vi "Receive Messages.vi"(6 "Wait Time":i32=-1, 8 "error in (no error)":errorcluster, 9 "Visibility Timeout":i32, 10 "Max Number of Messages":i32=1, 11 "SQS in":refnum<class "Queue.lvclass">) -> (0 "error out":errorcluster, 2 "Messages":T1[](array[typedef]), 3 "SQS out":refnum<class "Queue.lvclass">)   [LabVIEW 2015, in "NI_AWS_SQS.lvlib" / "Queue.lvclass"]
doc: "Retrieves one or more messages (up to 10), from the specified queue. Using the Wait Time parameter enables long-poll support. For more information, see Amazon SQS Long Polling in the Amazon SQS Developer Guide.\n\nShort poll is the default behavior where a weighted random set of machines is sampled on a ReceiveMessage call. Thus, only the messages on the sampled machines are returned. If the number of messages in the queue is small (fewer than 1,000), you most likely get fewer messages than you requested per ReceiveMessage call. If the number of messages in the queue is extremely small, you might not receive any messages in a particular ReceiveMessage response. If this happens, repeat the request.\n\nFor each message returned, the response includes the following:\n\nThe message body.\nAn MD5 digest of the message body. For information on MD5, see RFC1321.\nThe MessageId you received when you sent the message to the queue.\nThe receipt handle.\nThe message attributes.\nAn MD5 digest of the message attributes.\nThe receipt handle is the identifier you must provide when deleting the message. For more information, see Queue and Message Identifiers in the Amazon SQS Developer Guide.\n\nYou can provide the VisibilityTimeout parameter in your request. The parameter is applied to the messages that Amazon SQS returns in the response. If you don't include the parameter, the overall visibility timeout for the queue is used for the returned messages. For more information, see Visibility Timeout in the Amazon SQS Developer Guide.\n\nA message that isn't deleted or a message whose visibility isn't extended before the visibility timeout expires counts as a failed receive. Depending on the configuration of the queue, the message might be sent to the dead letter queue.\n\nNote\nIn the future, new attributes might be added. If you write code that calls this action, we recommend that you structure your code so that it can handle new attributes gracefully."
uses:
  Queue.lvclass
  Message.ctl
  Message Attribute Value Pair.ctl
  Message Attribute.ctl
  Custom Attribute.ctl
  Custom Attribute Type.ctl
  Core/HTTP Request/Name Value Pair.ctl
  Core/HTTP Request/Request Options.ctl
  Core/HTTP Request/Region handling.ctl
  Core/HTTP Request/URL formatting.ctl
  Queue.lvclass/Queue.ctl
  Read Account Number.vi
  Read Name.vi
  Core/HTTP Request/HTTP Request.lvclass
  XML Parsing/NI_XML Parsing.lvlib
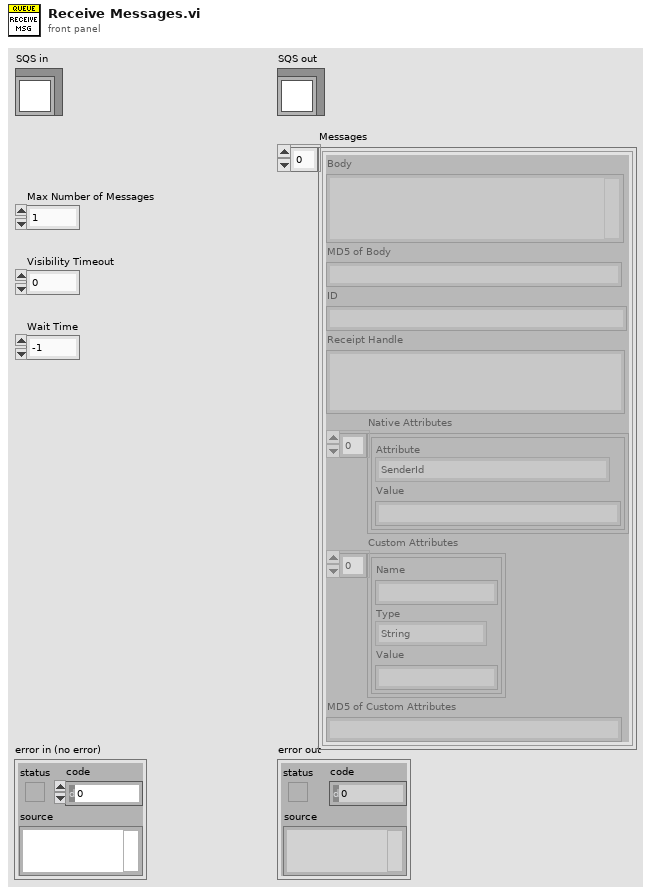
[diagram p1: front panel]
types:
  T1 = typedef "NI_AWS_SQS.lvlib/Queue.lvclass/Message.ctl" = cluster{"Body":string, "MD5 of Body":string, "ID":string, "Receipt Handle":string, "Native Attributes":T2[], "Custom Attributes":T4[], "MD5 of Custom Attributes":string}
  T2 = typedef "NI_AWS_SQS.lvlib/Queue.lvclass/Message Attribute Value Pair.ctl" = cluster{"Attribute":T3, "Value":string}
  T3 = typedef "NI_AWS_SQS.lvlib/Queue.lvclass/Message Attribute.ctl" = enum16{"SenderId", "SentTimestamp", "ApproximateReceiveCount", "ApproximateFirstReceiveTimestamp"}
  T4 = typedef "NI_AWS_SQS.lvlib/Queue.lvclass/Custom Attribute.ctl" = cluster{"Name":string, "Type":T5, "Value":string}
  T5 = typedef "NI_AWS_SQS.lvlib/Queue.lvclass/Custom Attribute Type.ctl" = enum16{"String", "Number", "Binary"}
  T6 = typedef "NI_AWS_Core.lvlib/HTTP Request.lvclass/Name Value Pair.ctl" = cluster{"name":string, "value":string}
  T7 = typedef "NI_AWS_Core.lvlib/HTTP Request.lvclass/Request Options.ctl" = cluster{"request headers":T6[], "request parameters":T6[], "request body":string, "region handling":T8, "URL formatting":T9}
  T8 = typedef "NI_AWS_Core.lvlib/HTTP Request.lvclass/Region handling.ctl" = enum16{"use region everywhere", "use region (authentication only)", "use region (URL only)", "ignore region everwhere"}
  T9 = typedef "NI_AWS_Core.lvlib/HTTP Request.lvclass/URL formatting.ctl" = enum16{"region-", "region."}
  T10 = typedef "NI_AWS_Core.lvlib/HTTP Request.lvclass/Response.ctl" = cluster{"Headers":string, "Body":string}
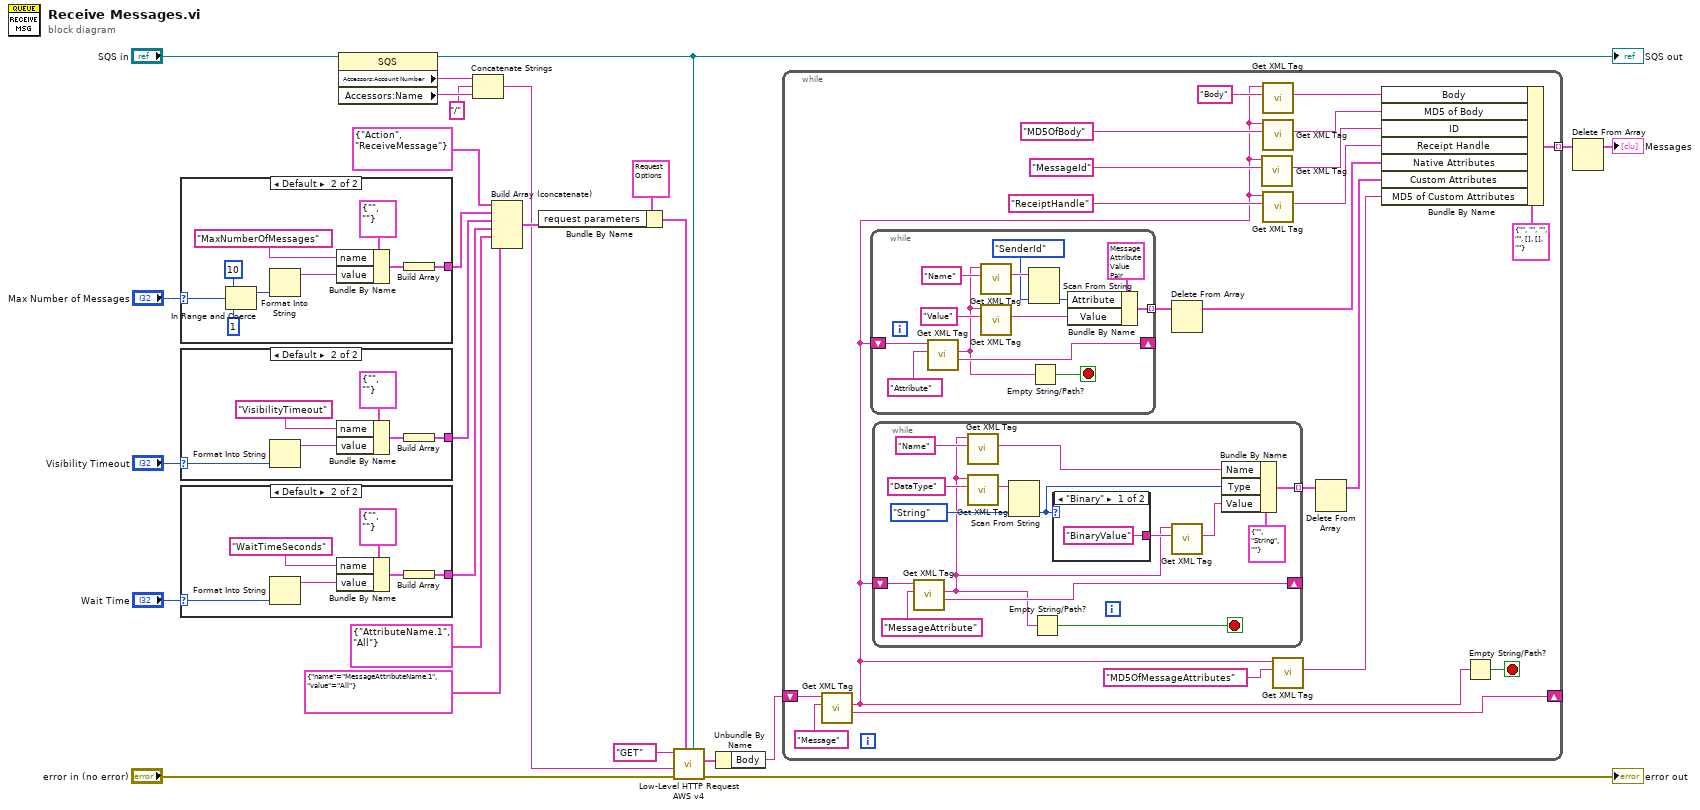
[diagram p0: block diagram]
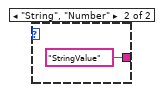
[diagram p2: hidden frame]
diagram:
  n1 = case shown="Default" "Max Number of Messages" {
    selector: "Max Number of Messages" -> [_ w32]
    tunnel: [_ w26] -> w10
    frame ..1 {
    }
    frame Default {
      n2 = In Range and Coerce(upper limit=10, x=w32, lower limit=1) -> (coerced(x)=w29:i32)  [unwired: 1 out]
      n3 = Format Into String(w29) -> (resulting string=w28:string)  [unwired: 3 in, 1 out]
      n4 = Bundle By Name(cluster=T6 {"name"="", "value"=""} ("element"), "name"="MaxNumberOfMessages", "value"=w28) -> (w27:T6)
      n5 = Build Array(w27) -> (w26:T6[])
    }
  }
  n6 = case shown="Default" "Visibility Timeout" {
    selector: "Visibility Timeout" -> [_ w40]
    tunnel: [_ w35] -> w8
    frame ..0 {
    }
    frame Default {
      n7 = Format Into String(w40) -> (resulting string=w37:string)  [unwired: 3 in, 1 out]
      n8 = Bundle By Name(cluster=T6 {"name"="", "value"=""} ("element"), "name"="VisibilityTimeout", "value"=w37) -> (w36:T6)
      n9 = Build Array(w36) -> (w35:T6[])
    }
  }
  n10 = case shown="Default" "Wait Time" {
    selector: "Wait Time" -> [_ w46]
    tunnel: [_ w41] -> w6
    frame ..-1 {
    }
    frame Default {
      n11 = Format Into String(w46) -> (resulting string=w43:string)  [unwired: 3 in, 1 out]
      n12 = Bundle By Name(cluster=T6 {"name"="", "value"=""} ("element"), "name"="WaitTimeSeconds", "value"=w43) -> (w42:T6)
      n13 = Build Array(w42) -> (w41:T6[])
    }
  }
  n14 = property class="SQS"(reference="SQS in") -> (reference out=w17:refnum<class "Queue.lvclass">, "Accessors:Account Number"=w16:string, "Accessors:Name"=w15:string)  [unwired: 1 in, 1 out]
  "SQS out" <- w17
  n15 = Concatenate Strings(w16, "/", w15) -> (w13:string)
  n16 = Build Array (concatenate)(T6 {"name"="Action", "value"="ReceiveMessage"} ("Cluster"), w10, w8, w6, T6 {"name"="AttributeName.1", "value"="All"} ("Cluster"), T6 {"name"="MessageAttributeName.1", "value"="All"} ("Cluster")) -> (w18:T6[])
  n17 = Bundle By Name(cluster=T7 {"request headers"=[], "request parameters"=[{"name"="Action", "value"="ListQueues"}], "request body"="", "region handling"=enum."use region everywhere", "URL formatting"=enum."region."} ("Request Options"), "request parameters"=w18) -> (w19:T7)
  n18 = call "Low-Level HTTP Request AWS v4.vi"("AWS Core"=w17, "Request Options"=w19, "error in (no error)"="error in (no error)", "URL Suffix"=w13, "HTTP-Verb"="GET") -> ("error out"=→"error out":errorcluster, "Response"=w22:T10)  [unwired: 4 in, 1 out]
  n19 = Unbundle By Name(w22) -> ("Body"=w21:string)
  n20 = while {
    shift-right: [w66] -> _
    shift-left: w21 -> [w67]
    tunnel: [w61] -> w4 mode=indexing
    stop <- w65 stop-if-true
    n21 = call "Get XML Tag.vi"("Tag name"="Message", "XML String in"=w67) -> ("Remaining string"=w66:string, "Tag value"=w49:string)  [unwired: 5 in, 3 out]
    n22 = while {
      shift-right: [w79] -> _
      shift-left: w49 -> [w80]
      tunnel: [w75] -> w53 mode=indexing
      stop <- w77 stop-if-true
      n23 = call "Get XML Tag.vi"("Tag name"="Attribute", "XML String in"=w80) -> ("Remaining string"=w79:string, "Tag value"=w72:string)  [unwired: 5 in, 3 out]
      n24 = call "Get XML Tag.vi"("Tag name"="Name", "XML String in"=w72) -> ("Tag value"=w69:string)  [unwired: 5 in, 4 out]
      n25 = call "Get XML Tag.vi"("Tag name"="Value", "XML String in"=w72) -> ("Tag value"=w71:string)  [unwired: 5 in, 4 out]
      n26 = Scan From String(input string=w69, default 1=Message_Attribute."SenderId" ("Attribute")) -> (output 1=w70:T3)  [unwired: 3 in, 3 out]
      n27 = Empty String/Path?(string/path=w72) -> (empty?=w77:bool)
      n28 = Bundle By Name(cluster=T2 {"Attribute"=enum."ApproximateFirstReceiveTimestamp", "Value"=""} ("Message Attribute Value Pair"), "Attribute"=w70, "Value"=w71) -> (w75:T2)
    }
    n29 = while {
      shift-right: [w94] -> _
      shift-left: w49 -> [w95]
      tunnel: [w91] -> w51 mode=indexing
      stop <- w92 stop-if-true
      n30 = call "Get XML Tag.vi"("Tag name"="MessageAttribute", "XML String in"=w95) -> ("Remaining string"=w94:string, "Tag value"=w81:string)  [unwired: 5 in, 3 out]
      n31 = call "Get XML Tag.vi"("Tag name"="Name", "XML String in"=w81) -> ("Tag value"=w87:string)  [unwired: 5 in, 4 out]
      n32 = call "Get XML Tag.vi"("Tag name"="DataType", "XML String in"=w81) -> ("Tag value"=w86:string)  [unwired: 5 in, 4 out]
      n33 = Scan From String(input string=w86, default 1=Custom_Attribute_Type."String" ("Custom Attribute Type")) -> (output 1=w84:T5)  [unwired: 3 in, 3 out]
      n34 = Empty String/Path?(string/path=w81) -> (empty?=w92:bool)
      n35 = case shown="\"Binary\"" w84 {
        tunnel: ["BinaryValue" "StringValue"] -> w83
        frame "Binary" {
        }
        frame "String", "Number" {
        }
      }
      n36 = call "Get XML Tag.vi"("Tag name"=w83, "XML String in"=w81) -> ("Tag value"=w82:string)  [unwired: 5 in, 4 out]
      n37 = Bundle By Name(cluster=T4 {"Name"="", "Type"=enum."String", "Value"=""} ("Custom Attribute"), "Name"=w87, "Type"=w84, "Value"=w82) -> (w91:T4)
    }
    n38 = Delete From Array(array=w53) -> (array with subset deleted=w52:T2[])  [unwired: 2 in, 1 out]
    n39 = call "Get XML Tag.vi"("Tag name"="MessageId", "XML String in"=w49) -> ("Tag value"=w57:string)  [unwired: 5 in, 4 out]
    n40 = call "Get XML Tag.vi"("Tag name"="Body", "XML String in"=w49) -> ("Tag value"=w58:string)  [unwired: 5 in, 4 out]
    n41 = call "Get XML Tag.vi"("Tag name"="MD5OfBody", "XML String in"=w49) -> ("Tag value"=w60:string)  [unwired: 5 in, 4 out]
    n42 = call "Get XML Tag.vi"("Tag name"="ReceiptHandle", "XML String in"=w49) -> ("Tag value"=w54:string)  [unwired: 5 in, 4 out]
    n43 = call "Get XML Tag.vi"("Tag name"="MD5OfMessageAttributes", "XML String in"=w49) -> ("Tag value"=w48:string)  [unwired: 5 in, 4 out]
    n44 = Delete From Array(array=w51) -> (array with subset deleted=w50:T4[])  [unwired: 2 in, 1 out]
    n45 = Bundle By Name(cluster=T1 {"Body"="", "MD5 of Body"="", "ID"="", "Receipt Handle"="", "Native Attributes"=[], "Custom Attributes"=[], "MD5 of Custom Attributes"=""} ("Message"), "Body"=w58, "MD5 of Body"=w60, "ID"=w57, "Receipt Handle"=w54, "Native Attributes"=w52, "Custom Attributes"=w50, "MD5 of Custom Attributes"=w48) -> (w61:T1)
    n46 = Empty String/Path?(string/path=w49) -> (empty?=w65:bool)
  }
  n47 = Delete From Array(array=w4) -> (array with subset deleted=→"Messages":T1[])  [unwired: 2 in, 1 out]
